vi "File explorer.vi"(0 "IP Address":string) -> ()   [LabVIEW 2017]
uses:
  <vilib>/WebDAVClient/Advanced/SessionHandle.ctl
  <vilib>/WebDAVClient/Advanced/Get File.vi
  <vilib>/WebDAVClient/NI_WebDAV.lvlib
panel:
  out "Close":bool
  in  "Stop":bool
  in  "Directory Listing":i32(listbox)=-1
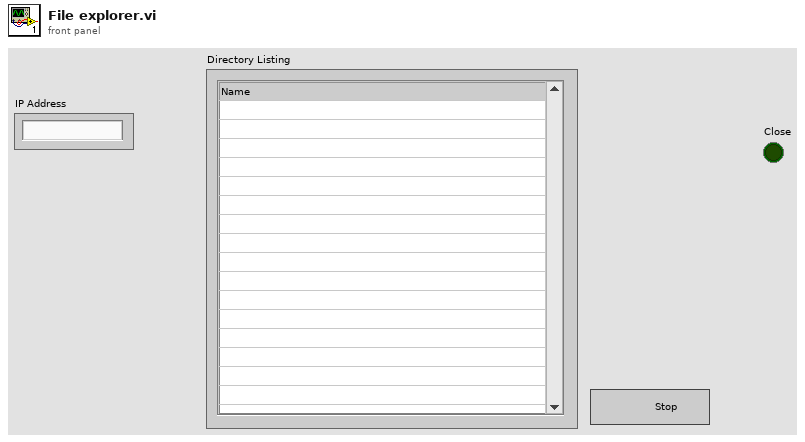
[diagram p1: front panel]
types:
  T1 = typedef "NI_WebDAV.lvlib/SessionHandle.ctl" = refnum<k1>
  T2 = typedef "NI_WebDAV.lvlib/FileInfo.ctl" = cluster{"type":string, "size":u64, "last modification":timestamp, "display name":string, "uri":string}
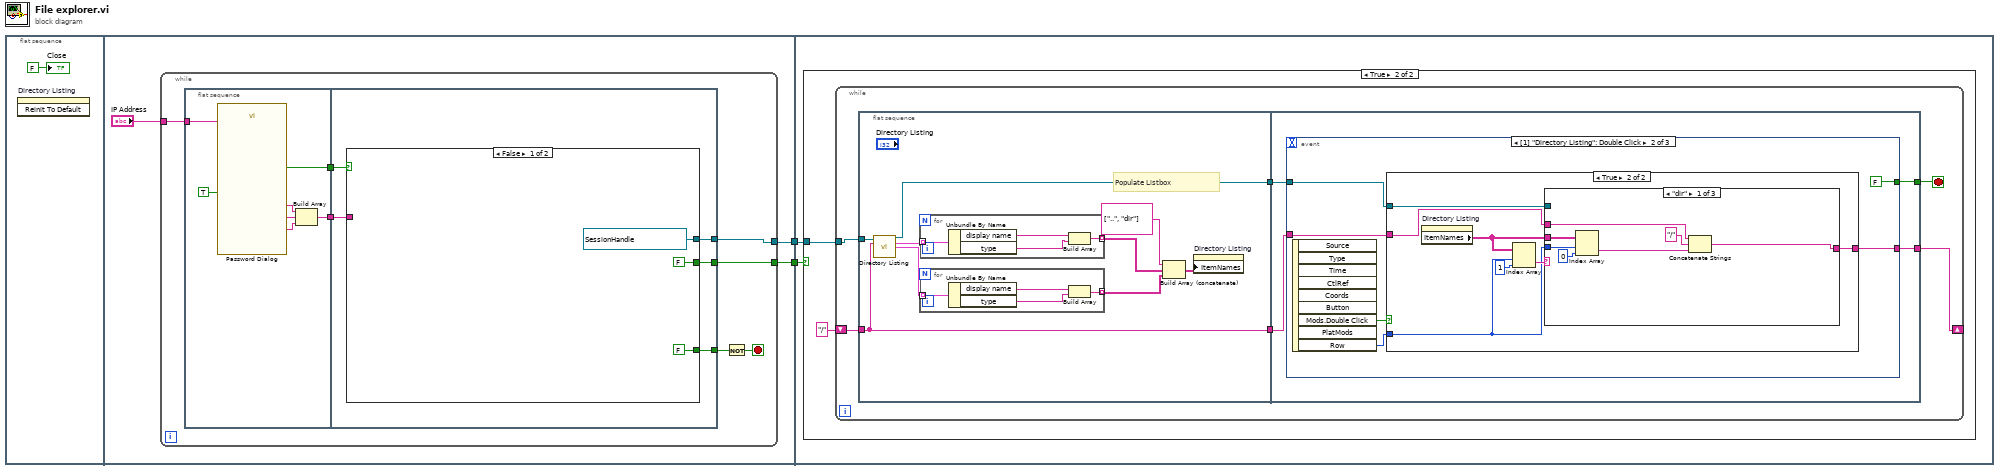
[diagram p0: block diagram]
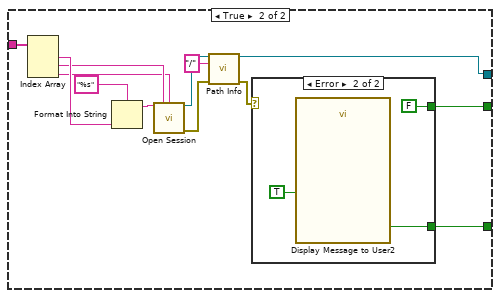
[diagram p2: hidden frame]
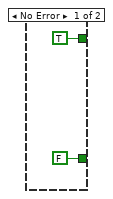
[diagram p3: hidden frame]
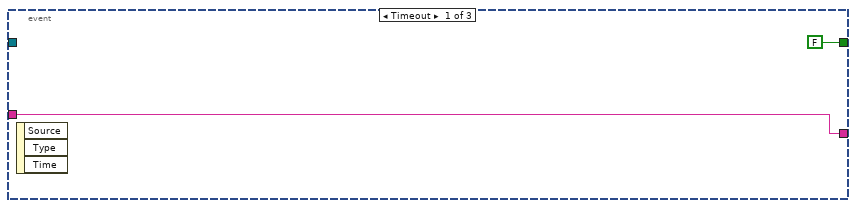
[diagram p5: hidden frame]
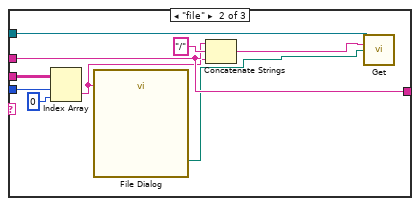
[diagram p7: hidden frame]
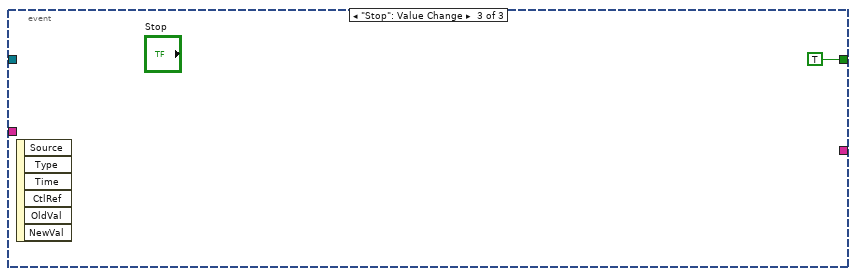
[diagram p9: hidden frame]
diagram:
  n1 = flat-sequence {
    tunnel: [w5] -> w2
    tunnel: [w4] -> w1
    tunnel: w2 -> [w48]
    tunnel: w1 -> [w47]
    frame #0 {
      n2 = invoke on="Directory Listing" class="MCListbox (strict)" method="Reinit To Default"() -> ()  [unwired: 3 in, 3 out]
      "Close" <- FALSE ("Close")
    }
    frame #1 {
      n3 = while {
        tunnel: "IP Address" -> [w12]
        tunnel: [w8] -> w5
        tunnel: [w7] -> w4
        stop <- w10 stop-if-true
        n4 = flat-sequence {
          tunnel: [w16] -> w13
          tunnel: w12 -> [w15]
          tunnel: [w14] -> w11
          tunnel: w13 -> [w25]
          tunnel: [w24] -> w9
          tunnel: w11 -> [w23]
          tunnel: [w22] -> w8
          tunnel: [w21] -> w7
          frame #0 {
            n5 = call "Password Dialog.vi"("Enable"=TRUE, "IP Placeholder"=w15) -> ("Password"=w17:string, "Username"=w18:string, "IP address"=w19:string, "OK"=w14:bool)  [unwired: 13 in, 1 out]
            n6 = Build Array(w19, w18, w17) -> (w16:string[])
          }
          frame #1 {
            n7 = case shown="False" w23 {
              tunnel: w25 -> [_ w41]
              tunnel: [FALSE ("Retry") w39] -> w24
              tunnel: [FALSE ("Retry") w33] -> w22
              tunnel: [w26 w29] -> w21
              frame False {
                w26 = T1 refnum items=["Session NI_WebDAV"] ("session handle out")
              }
              frame True {
                n8 = Index Array(array=w41) -> (element #1=w40:string, element #2=w32:string, element #3=w31:string)  [unwired: 3 in]
                n9 = Format Into String(format string="%s", w40) -> (resulting string=w38:string)  [unwired: 2 in, 1 out]
                n10 = call <vilib>:"Open Session.vi"("host uri prefix"=w38, "username"=w32, "password"=w31) -> ("session handle out"=w37:T1, "error out"=w36:errorcluster)  [unwired: 11 in]
                n11 = call <vilib>:"Path Info.vi"("session handle"=w37, "relative uri"="/", "error in (no error)"=w36) -> ("session handle out"=w29:T1, "error out"=w34:errorcluster)  [unwired: 9 in, 2 out]
                n12 = case shown="Error" w34 {
                  tunnel: [FALSE ("Retry") w45] -> w39
                  tunnel: [TRUE FALSE] -> w33
                  frame No Error {
                  }
                  frame Error {
                    n13 = call "Display Message to User2"("Enable"=TRUE) -> ("Retry"=w45:bool)  [unwired: 9 in, 1 out]
                  }
                }
              }
            }
          }
        }
        n14 = Not(x=w9) -> (.not. x?=w10:bool)
      }
    }
    frame #2 {
      n15 = case shown="True" w48 {
        tunnel: w47 -> [_ w49]
        frame False {
        }
        frame True {
          n16 = while {
            shift-right: [w53] -> _
            shift-left: "/" -> [w56]
            tunnel: w49 -> [w51]
            stop <- w52 stop-if-true
            n17 = flat-sequence {
              tunnel: w56 -> [w62]
              tunnel: [w63] -> w55
              tunnel: [w62] -> w54
              tunnel: w51 -> [w61]
              tunnel: w55 -> [w77]
              tunnel: w54 -> [w76]
              tunnel: [w75] -> w53
              tunnel: [w74] -> w52
              frame #0 {
                # "Populate Listbox"
                n18 = call <vilib>:"Directory Listing.vi"("session handle"=w61, "relative uri"=w62) -> ("session handle out"=w63:T1, "directory list"=w59:T2[], "file list"=w58:T2[])  [unwired: 10 in, 1 out]
                n19 = for {
                  tunnel: [w72] -> w60 mode=indexing
                  tunnel: w59 -> [w70] mode=indexing
                  n20 = Unbundle By Name(w70) -> ("display name"=w73:string, "type"=w71:string)
                  n21 = Build Array(w73, w71) -> (w72:string[])
                }
                n22 = for {
                  tunnel: [w68] -> w57 mode=indexing
                  tunnel: w58 -> [w66] mode=indexing
                  n23 = Unbundle By Name(w66) -> ("display name"=w69:string, "type"=w67:string)
                  n24 = Build Array(w69, w67) -> (w68:string[])
                }
                n25 = Build Array (concatenate)(string[] ["..", "dir"], w60, w57) -> (w65:string[][])
                n26 = property on="Directory Listing" class="MCListbox (strict)"("ItemNames"=w65) -> ()  [unwired: 2 in, 2 out]
              }
              frame #1 {
                n27 = event shown="[1] \"Directory Listing\": Double Click" {
                  selector: _ -> [_ _ _]
                  dyn-events: _ -> [_ _ _]
                  timeout: _ -> [_ _ _]
                  tunnel: w76 -> [w79 w83 _]
                  tunnel: [w79 w82 _] -> w75
                  tunnel: w77 -> [_ w81 _]
                  tunnel: [FALSE FALSE TRUE] -> w74
                  event Timeout {
                    n28 = event-data() -> ()  [unwired: 1 in, 3 out]
                  }
                  event "Directory Listing": Double Click {
                    n29 = event-data() -> ("Mods.Double Click"=w85:bool, "Row"=w84:i32)  [unwired: 1 in, 7 out]
                    n30 = case shown="True" w85 {
                      tunnel: w83 -> [w86 w88]
                      tunnel: w84 -> [_ w89]
                      tunnel: [w86 w91] -> w82
                      tunnel: w81 -> [_ w87]
                      frame False {
                      }
                      frame True {
                        n31 = property on="Directory Listing" class="MCListbox (strict)"() -> ("ItemNames"=w90:string[][])  [unwired: 2 in, 2 out]
                        n32 = Index Array(array=w90, index (row)=w89, index (col)=1 ("disabled index (col)")) -> (element=w92:string)
                        n33 = case shown="\"dir\"" w92 {
                          tunnel: [w99 w105 w110] -> w91
                          tunnel: w90 -> [w98 w107 _]
                          tunnel: w89 -> [w96 w108 _]
                          tunnel: w88 -> [w94 w105 w110]
                          tunnel: w87 -> [_ w103 _]
                          frame "dir" {
                            n34 = Index Array(array=w98, index (row)=w96, index (col)=0 ("disabled index (col)")) -> (element=w95:string)
                            n35 = Concatenate Strings(w94, "/" ("string"), w95) -> (w99:string)
                          }
                          frame "file" {
                            n36 = Index Array(array=w107, index (row)=w108, index (col)=0 ("disabled index (col)")) -> (element=w104:string)
                            n37 = call "File Dialog"("default name"=w104) -> ("selected path"=w101:path)  [unwired: 11 in, 3 out]
                            n38 = Concatenate Strings(w105, "/" ("string"), w104) -> (w102:string)
                            n39 = call-poly <vilib>:"Get.vi"("session handle"=w103, "relative uri"=w102, "local file path"=w101) -> ()  [unwired: 10 in, 3 out]
                          }
                          frame "link", "unknown", Default {
                          }
                        }
                      }
                    }
                  }
                  event "Stop": Value Change {
                    n40 = event-data() -> ()  [unwired: 1 in, 6 out]
                  }
                }
              }
            }
          }
        }
      }
    }
  }
